vi "Install LabVIEW Support Legacy.vi"() -> ()   [LabVIEW 2020, in "LMH-LINX.lvlib"]
uses:
  LMH-LINX.lvlib
  Install LV Events.ctl
  Target Management/Install LV Data.ctl
  Target Management/Target Info.ctl
  Target Management/NIC Info.ctl
  Target Management/NIC Mode.ctl
  Target Management/Status FGV States.ctl
  <vilib>/Platform/browser.llb/Open URL in Default Browser (path).vi
  Toolbox/LMH-Toolbox.lvlib
panel:
  in  "Finish":bool
  in  "Example":bool
  in  "Install":bool
  in  "Password":string="raspberry"
  in  "Username":string="pi"
  in  "Hostname or IP":string="raspberrypi"
  out "Live Status":string
  in  "View Log":bool
  out "EULA Link":string="here"
  in  "Connect":bool
  out "Event Handler Iterations":i32
  out "Detailed Log":string
  out "Status Log":string
  out "Error Out":errorcluster
  # "LINX\nInstall LabVIEW Suport Wizard"
  # "This wizard will install LabVIEW support on BeagleBone Black or Raspberry Pi 2.\n\n1. Ensure the target is powered on, connected to this computer, and that the target has internet access.\n2. Enter the target's hostname or IP address.\n3. Enter the username and password for an account with sudo privileges on the target.\n          BBB defaults to 'root' and no password.\n          RPI2 running Raspbian defaults to 'pi' and 'raspberry'."
  # "The software installed by this wizard may be deployed on your hardware targets solely for your personal, \nnon-commercial use. Software is provided AS IS and with NO EXPRESS OR IMPLIED WARRANTIES.  \nThe full terms of the license can be found         ."
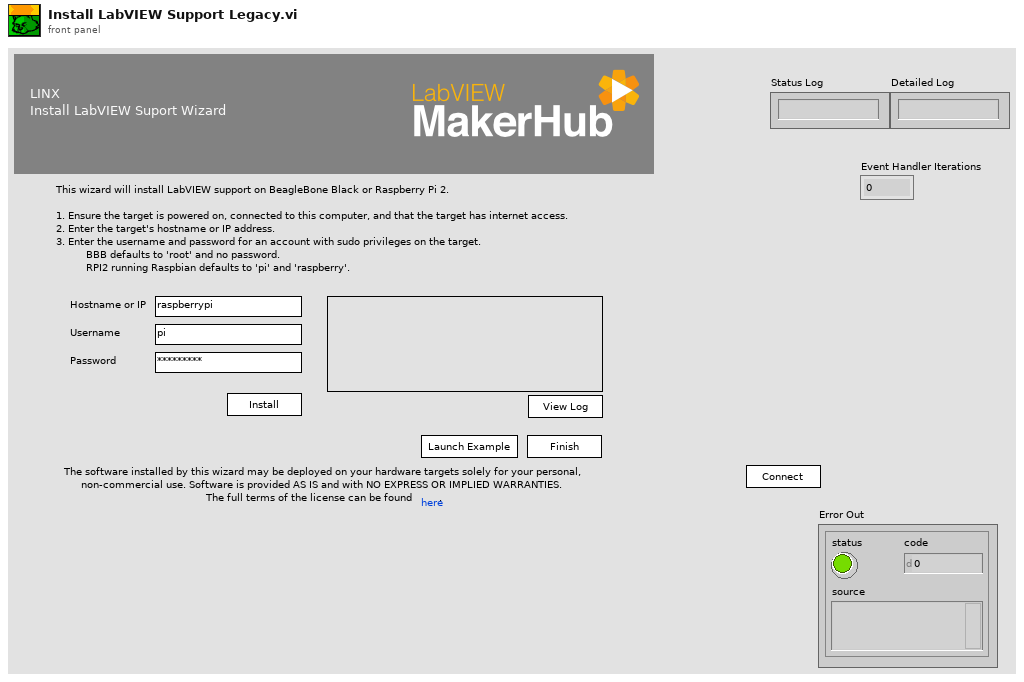
[diagram p1: front panel]
types:
  T1 = typedef "LMH-LINX.lvlib/Install LV Data.ctl" = cluster{"SSH Session":refnum<k1>, "Status Log":string, "Detailed Log":string, "Credentials":cluster{"Hostname or IP":string, "Username":string, "Password":string}, "Target Info":T2, "Reboot Required?":bool}
  T2 = typedef "LMH-LINX.lvlib/Target Info.ctl" = cluster{"OS Version":string, "CPU":string, "Systemd Version":string, "Internet Access":bool, "Device Type":string, "LV Installed Ver":string, "LV Available Ver":string, "LV Upgrade Available":bool, "Hostname":string, "NIC Info":T3[]}
  T3 = typedef "LMH-LINX.lvlib/NIC Info.ctl" = cluster{"Name":string, "NIC Mode":T4, "Configured":bool, "Config IP address":string, "Config Subnet mask":string, "Config Network":string, "Config gateway":string, "Wifi":bool, "SSID":string, "Password":string, "Configuration":string, "Current IP address":string, "Current Subnet mask":string, "Current gateway":string, "Current Network":string}
  T4 = typedef "LMH-LINX.lvlib/NIC Mode.ctl" = enum16{"DHCP", "Static", "Loopback"}
  T5 = typedef "LMH-LINX.lvlib/Install LV Events.ctl" = enum16{"Idle", "Connect", "Interrogate Device", "Pre Install", "Add MakerHub Feed", "Update Package Index", "Install LV", "Start LV", "Launch Example", "View Log", "Exit", "Update Hostname", "Menu: Target", "Menu: Install Software", "Menu: Network Settings", "Menu: Target Info", "NIC Select Change", "Menu: Network Settings Save", "Menu: Network Settings Cancel", "Menu: Cancel All"}
  T6 = typedef "LMH-LINX.lvlib/Status FGV States.ctl" = enum16{"Init", "Append", "Append History Only", "Set", "Get"}
  T7 = typedef "LMH-LINX.lvlib/Target Compatibility Warnings.ctl" = cluster{"Warning?":bool, "Details":string, "Help URL":string, "Fix It Button Name":string, "Fix It VI Ref":refnum<vi>}
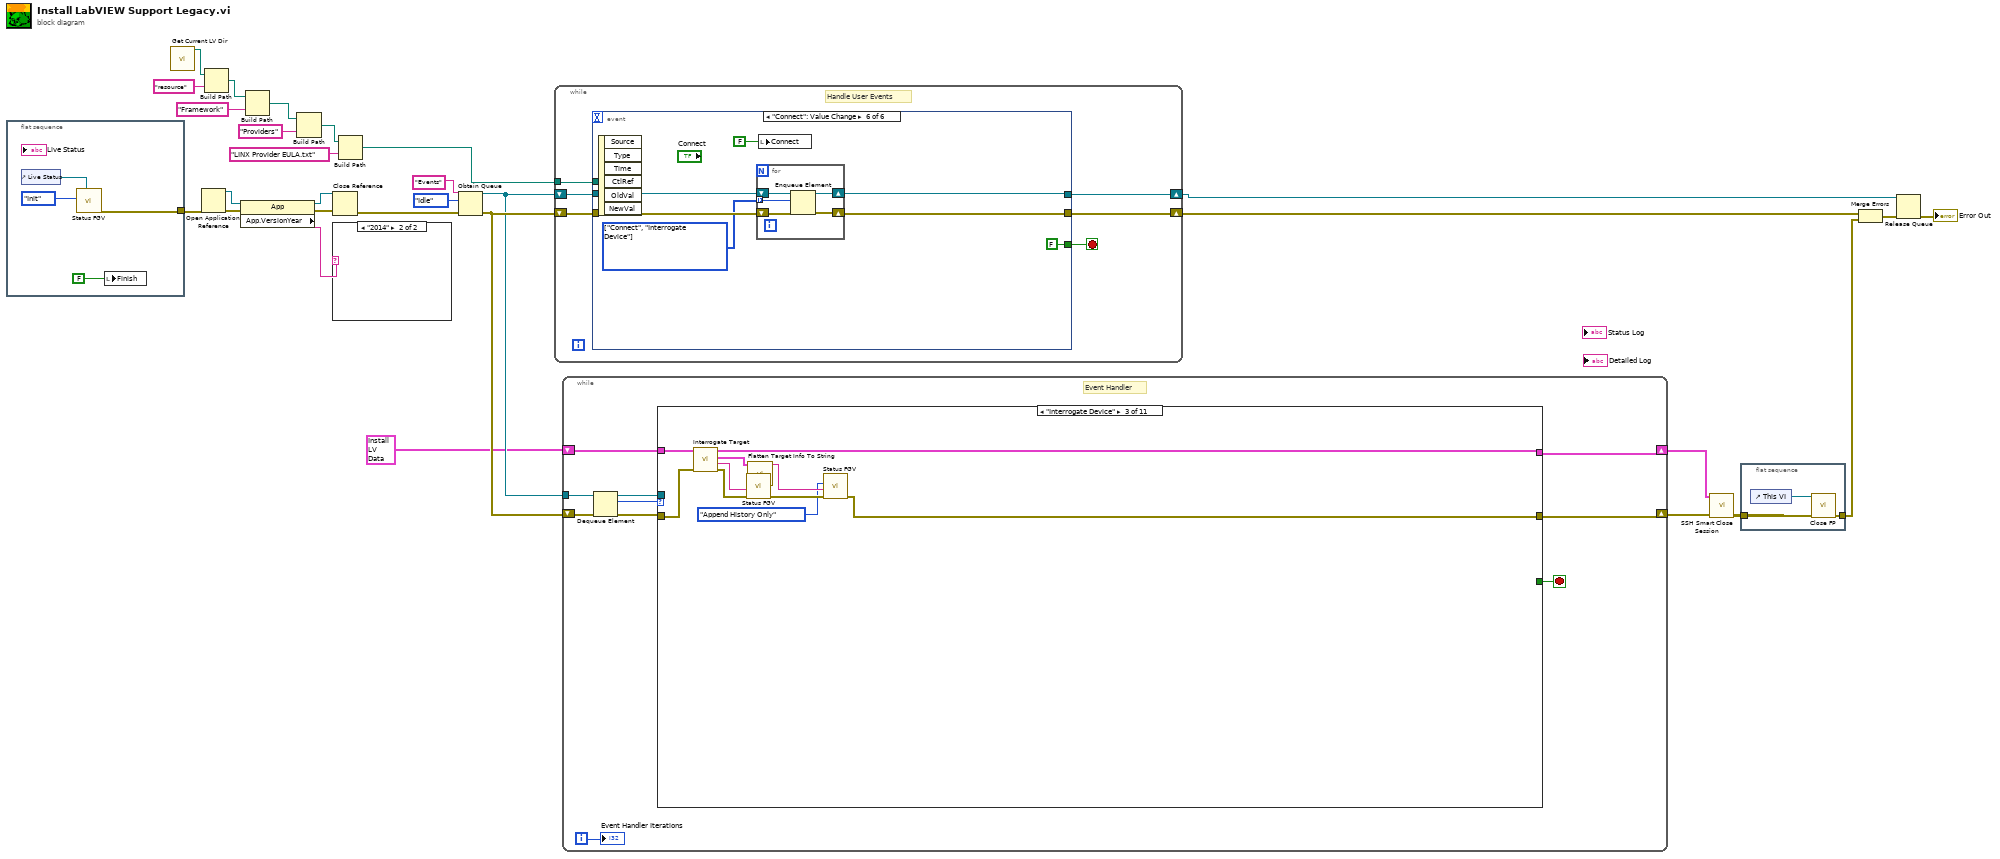
[diagram p0: block diagram]
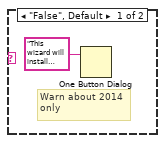
[diagram p2: hidden frame]
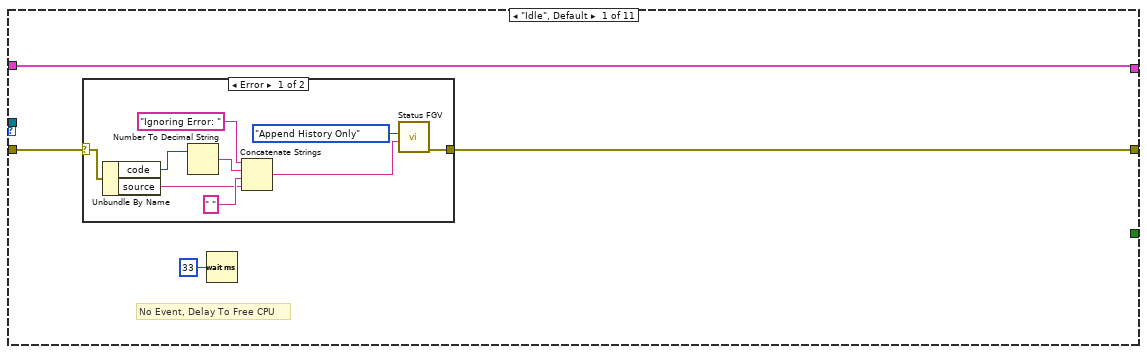
[diagram p3: hidden frame]
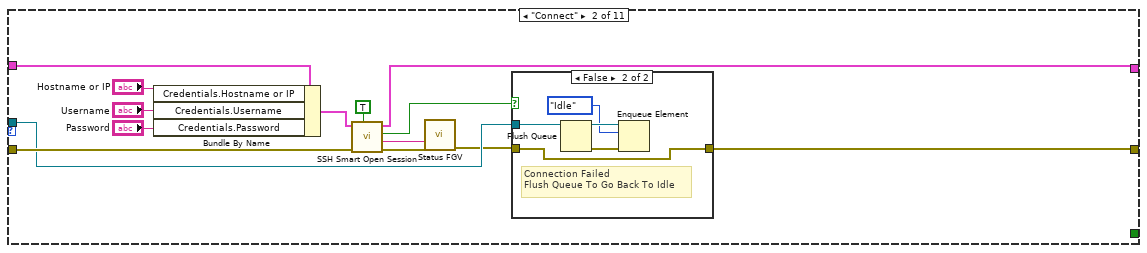
[diagram p5: hidden frame]
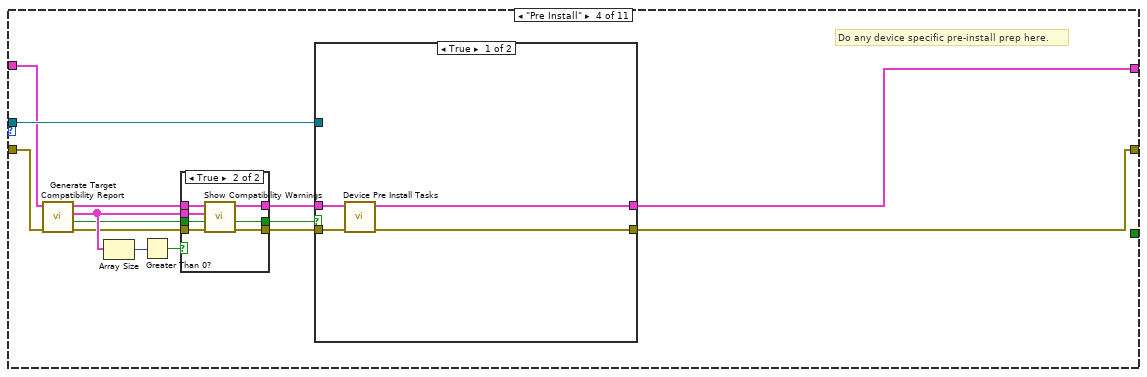
[diagram p7: hidden frame]
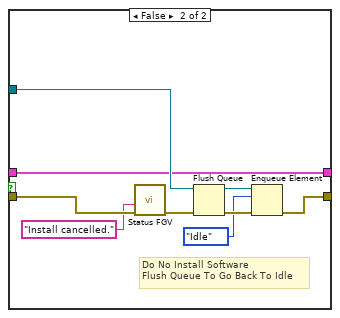
[diagram p8: hidden frame]
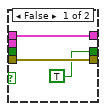
[diagram p9: hidden frame]
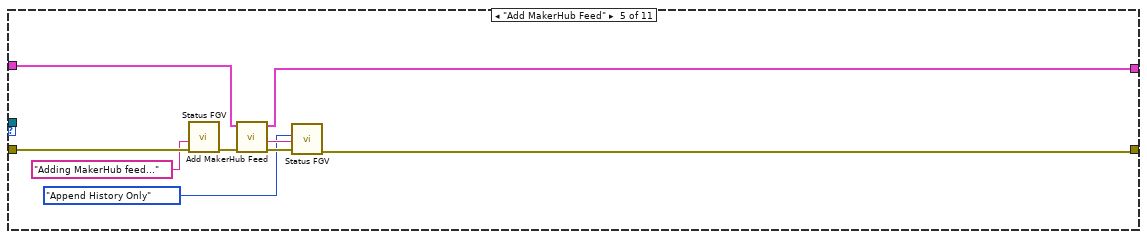
[diagram p10: hidden frame]
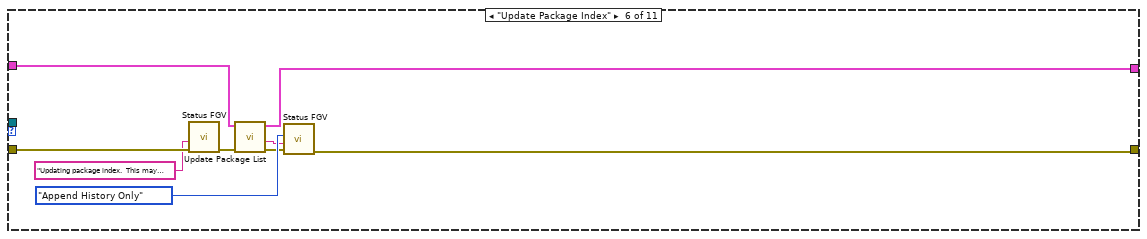
[diagram p11: hidden frame]
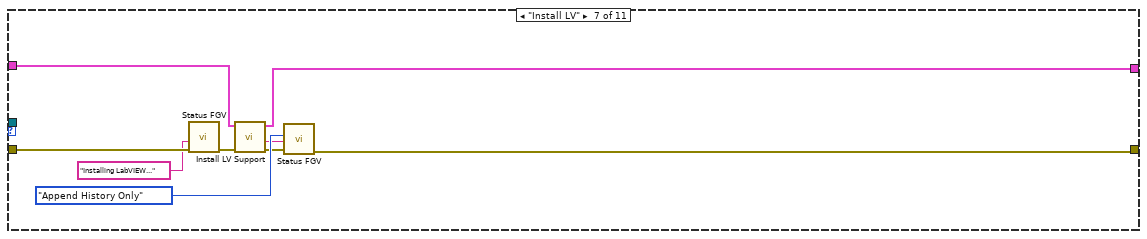
[diagram p12: hidden frame]
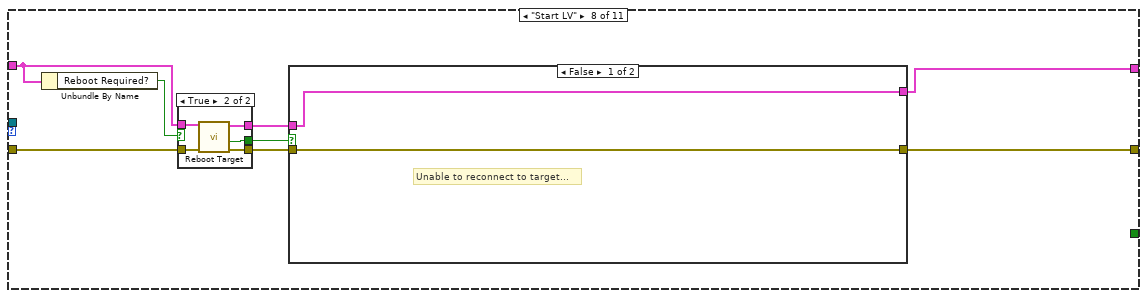
[diagram p13: hidden frame]
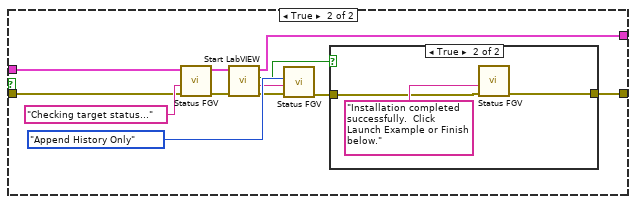
[diagram p14: hidden frame]
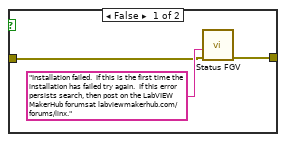
[diagram p15: hidden frame]
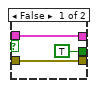
[diagram p16: hidden frame]
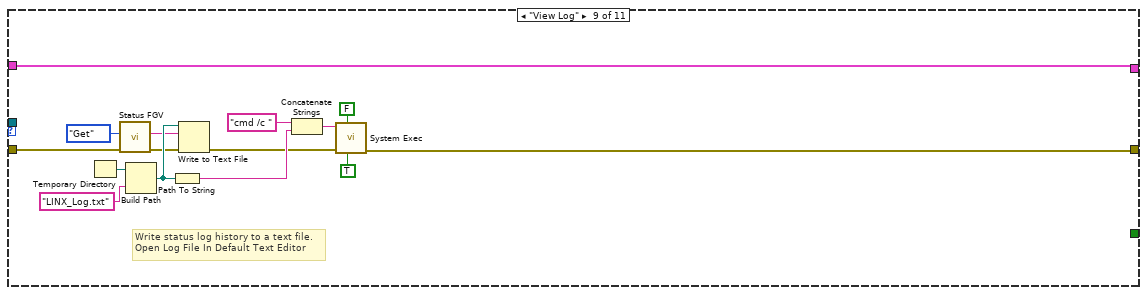
[diagram p17: hidden frame]
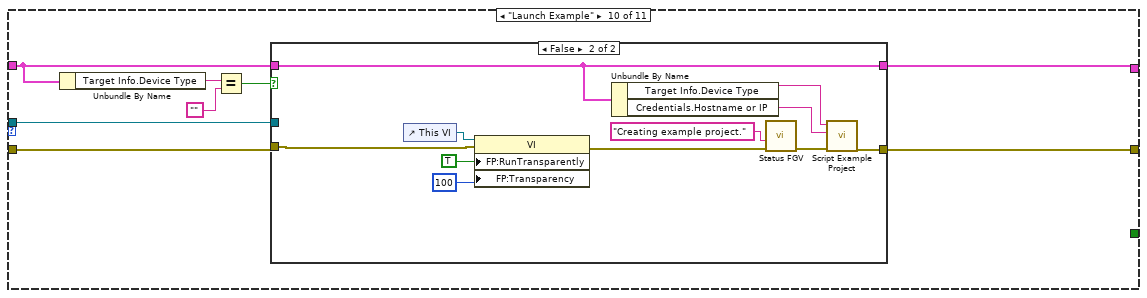
[diagram p18: hidden frame]
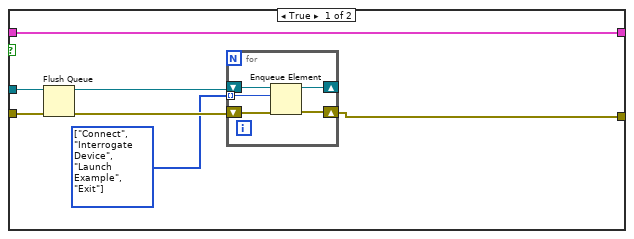
[diagram p19: hidden frame]
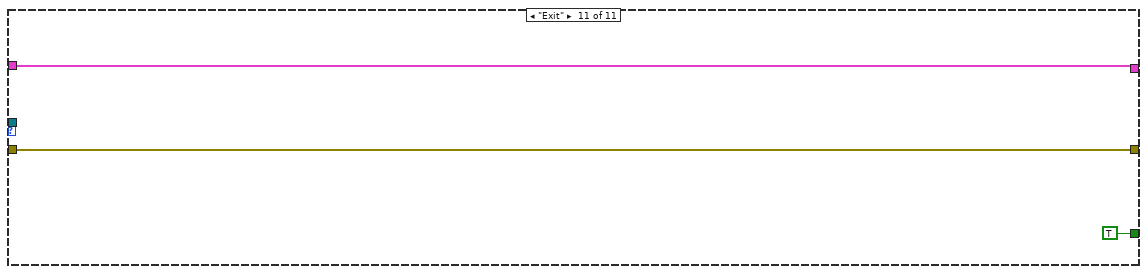
[diagram p20: hidden frame]
diagram:
  n1 = flat-sequence {
    tunnel: [w30] -> w6
    frame #0 {
      n2 = control-ref of="Live Status"() -> (w32:refnum<vi>)
      n3 = call "Status FGV.vi"("Live Status Ref"=w32, "Status FGV State"=Status_FGV_States."Init") -> ("Error Out"=w30:errorcluster)  [unwired: 7 in, 2 out]
      n4 = local write "Finish"(FALSE ("Stop Button")) -> ()
    }
  }
  n5 = call "Get Current LV Dir.vi"() -> ("This LV Directory"=w29:path)  [unwired: 10 in, 1 out]
  n6 = Open Application Reference(8:w6) -> (0:w19:errorcluster, 3:w16:refnum<vi>)  [unwired: 3 in]
  n7 = Build Path(base path=w29, name or relative path="resource") -> (appended path=w22:path)
  n8 = property class="App"(reference=w16, error in=w19) -> (reference out=w17:refnum<vi>, error out=w18:errorcluster, "App.VersionYear"=w20:string)
  n9 = Build Path(base path=w22, name or relative path="Framework") -> (appended path=w23:path)
  n10 = Build Path(base path=w23, name or relative path="Providers") -> (appended path=w24:path)
  n11 = Close Reference(reference=w17, error in (no error)=w18) -> (error out=w14:errorcluster)
  n12 = case shown="\"2014\"" w20 {
    frame "False", Default {
      # "Warn about 2014\nonly"
      n13 = One Button Dialog(message="This wizard will install LabVIEW 2014 support to the target device.  \nYou will only be able to connect to and use the device from LabVIEW 2014.") -> ()  [unwired: 1 in, 1 out]
    }
    frame "2014" {
    }
  }
  n14 = Build Path(base path=w24, name or relative path="LINX Provider EULA.txt") -> (appended path=w21:path)
  n15 = Obtain Queue(name (unnamed)="Events", element data type=Install_LV_Events."Idle" ("Install LV Support State"), error in (no error)=w14) -> (queue out=w12:refnum<queue>, error out=w13:errorcluster)  [unwired: 2 in, 1 out]
  n16 = while {
    shift-right: [w39] -> w2
    shift-left: w13 -> [w40]
    tunnel: w21 -> [w37]
    shift-right: [w36] -> w8
    shift-left: w12 -> [w35]
    stop <- w38 stop-if-true
    # "Handle User Events"
    n17 = event shown="[5] \"Connect\": Value Change" {
      selector: _ -> [_ _ _ _ _ _]
      dyn-events: _ -> [_ _ _ _ _ _]
      timeout: _ -> [_ _ _ _ _ _]
      tunnel: [w45 w64 w72 w76 w81 w92] -> w39
      tunnel: w40 -> [w46 w65 w70 w77 w86 w91]
      tunnel: [FALSE TRUE FALSE FALSE TRUE FALSE] -> w38
      tunnel: w37 -> [_ _ w71 _ _ _]
      tunnel: [w43 w63 w68 w75 w82 w93] -> w36
      tunnel: w35 -> [w42 w62 w68 w74 w87 w94]
      event "Install": Value Change {
        w41 = T5[] [enum."Connect", enum."Interrogate Device", enum."Pre Install", enum."Add MakerHub Feed", enum."Update Package Index", enum."Install LV", enum."Start LV"] items=["Idle", "Connect", "Interrogate Device", "Pre Install", "Add MakerHub Feed", "Update Package Index", "Install LV", "Start LV", "Launch Example", "View Log", "Exit", "Update Hostname", "Menu: Target", "Menu: Install Software", "Menu: Network Settings", "Menu: Target Info", "NIC Select Change", "Menu: Network Settings Save", "Menu: Network Settings Cancel", "Menu: Cancel All"]
        n18 = event-data() -> ("NewVal"=w44:bool)  [unwired: 1 in]
        n19 = local write "Install"(FALSE ("Install")) -> ()
        n20 = case shown="True" w44 {
          tunnel: w46 -> [w50 w55]
          tunnel: [w50 w54] -> w45
          tunnel: [w49 w53] -> w43
          tunnel: w42 -> [w49 w52]
          tunnel: w41 -> [_ w51]
          frame False {
            # "Ignore Change \nto False"
          }
          frame True {
            n21 = for {
              shift-right: [w59] -> w54
              shift-left: w55 -> [w60]
              shift-right: [w58] -> w53
              shift-left: w52 -> [w57]
              tunnel: w51 -> [w56] mode=indexing
              n22 = Enqueue Element(queue=w57, element=w56, error in (no error)=w60) -> (queue out=w58:refnum<queue>, error out=w59:errorcluster)  [unwired: 1 in, 1 out]
            }
          }
        }
      }
      event "Finish": Value Change {
        n23 = event-data() -> ()  [unwired: 1 in, 6 out]
        n24 = local write "Finish"(FALSE ("Stop Button")) -> ()
        n25 = Enqueue Element(queue=w62, element=Install_LV_Events."Exit", error in (no error)=w65) -> (queue out=w63:refnum<queue>, error out=w64:errorcluster)  [unwired: 1 in, 1 out]
      }
      event "EULA Link": Mouse Up {
        n26 = event-data() -> ()  [unwired: 1 in, 1 out]
        n27 = call-poly <vilib>:"Open URL in Default Browser.vi"("error in (no error)"=w70, "path"=w71) -> ("error out"=w72:errorcluster)  [unwired: 4 in, 1 out]
      }
      event "View Log": Value Change {
        n28 = event-data() -> ()  [unwired: 1 in, 1 out]
        n29 = Enqueue Element(queue=w74, element=Install_LV_Events."View Log", error in (no error)=w77) -> (queue out=w75:refnum<queue>, error out=w76:errorcluster)  [unwired: 1 in, 1 out]
        n30 = local write "View Log"(FALSE ("View Log")) -> ()
      }
      event "Example": Value Change {
        n31 = event-data() -> ()  [unwired: 1 in, 6 out]
        n32 = Enqueue Element(queue=w87, element=Install_LV_Events."Launch Example" ("Install LV Support State"), error in (no error)=w86) -> (queue out=w83:refnum<queue>, error out=w84:errorcluster)  [unwired: 1 in, 1 out]
        n33 = local write "Example"(FALSE ("Launch Example")) -> ()
        n34 = Enqueue Element(queue=w83, element=Install_LV_Events."Exit" ("Install LV Support State"), error in (no error)=w84) -> (queue out=w82:refnum<queue>, error out=w81:errorcluster)  [unwired: 1 in, 1 out]
      }
      event "Connect": Value Change {
        w90 = T5[] [enum."Connect", enum."Interrogate Device"] items=["Idle", "Connect", "Interrogate Device", "Pre Install", "Add MakerHub Feed", "Update Package Index", "Install LV", "Start LV", "Launch Example", "View Log", "Exit", "Update Hostname", "Menu: Target", "Menu: Install Software", "Menu: Network Settings", "Menu: Target Info", "NIC Select Change", "Menu: Network Settings Save", "Menu: Network Settings Cancel", "Menu: Cancel All"]
        n35 = event-data() -> ()  [unwired: 1 in, 6 out]
        n36 = for {
          shift-right: [w100] -> w92
          shift-left: w91 -> [w101]
          shift-right: [w99] -> w93
          shift-left: w94 -> [w98]
          tunnel: w90 -> [w97] mode=indexing
          n37 = Enqueue Element(queue=w98, element=w97, error in (no error)=w101) -> (queue out=w99:refnum<queue>, error out=w100:errorcluster)  [unwired: 1 in, 1 out]
        }
        n38 = local write "Connect"(FALSE ("Interrogate")) -> ()
      }
    }
  }
  n39 = while {
    shift-right: [w110] -> w7
    shift-left: w13 -> [w108]
    tunnel: w12 -> [w109]
    shift-right: [w105] -> w1
    shift-left: T1 {"SSH Session"=refnum, "Status Log"="", "Detailed Log"="", "Credentials"={"Hostname or IP"="", "Username"="", "Password"=""}, "Target Info"={"OS Version"="", "CPU"="", "Systemd Version"="", "Internet Access"=FALSE, "Device Type"="", "LV Installed Ver"="", "LV Available Ver"="", "LV Upgrade Available"=FALSE, "Hostname"="", "NIC Info"=[]}, "Reboot Required?"=FALSE} ("Install LV Data") -> [w103]
    i -> [w104]
    stop <- w111 stop-if-true
    # "Event Handler"
    n40 = Dequeue Element(queue=w109, error in (no error)=w108) -> (queue out=w102:refnum<queue>, element=w106:T5, error out=w107:errorcluster)  [unwired: 1 in, 1 out]
    n41 = case shown="\"Interrogate Device\"" w106 {
      tunnel: [w112 w135 w146 w160 w195 w207 w216 w227 w263 w276 w302] -> w110
      tunnel: w107 -> [w113 w139 w155 w164 w201 w210 w219 w225 w258 w277 w302]
      tunnel: [_ _ _ _ _ _ _ _ _ _ TRUE] -> w111
      tunnel: [w114 w126 w147 w159 w193 w202 w211 w221 w261 w270 w301] -> w105
      tunnel: w103 -> [w114 w128 w148 w158 w194 w203 w212 w223 w261 w271 w301]
      tunnel: w102 -> [_ w136 _ w165 _ _ _ _ _ w272 _]
      frame "Idle", Default {
        # "No Event, Delay To Free CPU"
        n42 = case shown="Error" w113 {
          selector: w113 -> [w123 w125]
          tunnel: [w124 w125] -> w112
          frame Error {
            n43 = Unbundle By Name(w123) -> ("code"=w121:i32, "source"=w118:string)
            n44 = Number To Decimal String(number=w121) -> (decimal integer string=w120:string)  [unwired: 1 in]
            n45 = Concatenate Strings("Ignoring Error: " ("Status"), w120, " " ("string"), w118) -> (w117:string)
            n46 = call "Status FGV.vi"("Status"=w117, "Status FGV State"=Status_FGV_States."Append History Only") -> ("Error Out"=w124:errorcluster)  [unwired: 7 in, 2 out]
          }
          frame No Error {
          }
        }
        n47 = Wait (ms)(milliseconds to wait=u32 33) -> ()  [unwired: 1 out]
      }
      frame "Connect" {
        n48 = Bundle By Name(cluster=w128, "Credentials.Hostname or IP"="Hostname or IP", "Credentials.Username"="Username", "Credentials.Password"="Password") -> (w127:T1)
        n49 = call "SSH Smart Open Session.vi"("Force Reconnect?"=TRUE, "Error In"=w139, "Install LV Data in"=w127) -> ("Error Out"=w134:errorcluster, "Status"=w132:string, "Connected?"=w137:bool, "Install LV Data out"=w126:T1)  [unwired: 5 in]
        n50 = call "Status FGV.vi"("Error In"=w134, "Status"=w132) -> ("Error Out"=w133:errorcluster)  [unwired: 7 in, 2 out]
        n51 = case shown="False" w137 {
          tunnel: w136 -> [_ w145]
          tunnel: w133 -> [w140 w141]
          tunnel: [w140 w141] -> w135
          frame True {
          }
          frame False {
            # "Connection Failed\nFlush Queue To Go Back To Idle"
            n52 = Flush Queue(queue=w145) -> (queue out=w143:refnum<queue>, error out=w144:errorcluster)  [unwired: 1 in, 1 out]
            n53 = Enqueue Element(queue=w143, element=Install_LV_Events."Idle", error in (no error)=w144) -> ()  [unwired: 1 in, 3 out]
          }
        }
      }
      frame "Interrogate Device" {
        n54 = call "Interrogate Target.vi"("Error In"=w155, "Install LV Data"=w148) -> ("Error Out"=w154:errorcluster, "Status"=w153:string, "Target Info"=w152:T2, "Install LV Data"=w147:T1)  [unwired: 6 in]
        n55 = call "Status FGV.vi"("Error In"=w154, "Status"=w153) -> ("Error Out"=w150:errorcluster)  [unwired: 7 in, 2 out]
        n56 = call "Flatten Target Info To String.vi"("Target Info"=w152) -> ("Target Info String"=w151:string)  [unwired: 10 in]
        n57 = call "Status FGV.vi"("Error In"=w150, "Status"=w151, "Status FGV State"=Status_FGV_States."Append History Only") -> ("Error Out"=w146:errorcluster)  [unwired: 6 in, 2 out]
      }
      frame "Pre Install" {
        # "Do any device specific pre-install prep here."
        n58 = call "Generate Target Compatibility Report.vi"("Error In"=w164, "Install LV Data"=w158) -> ("Error Out"=w161:errorcluster, "Can Continue?"=w162:bool, "Warnings"=w163:T7[], "Install LV Data"=w157:T1)  [unwired: 6 in]
        n59 = Array Size(array=w163) -> (size(s)=w169:i32)
        n60 = Greater Than 0?(x=w169) -> (x > 0?=w168:bool)
        n61 = case shown="True" w168 {
          tunnel: [w185 w192] -> w167
          tunnel: [TRUE ("Continue?") w191] -> w166
          tunnel: w161 -> [w185 w190]
          tunnel: w163 -> [_ w189]
          tunnel: w162 -> [_ w188]
          tunnel: w157 -> [w183 w187]
          tunnel: [w183 w186] -> w156
          frame False {
          }
          frame True {
            n62 = call "Show Compatibility Warnings.vi"("Error In"=w190, "Can Continue?"=w188, "Warnings"=w189, "Install LV Data"=w187) -> ("Error Out"=w192:errorcluster, "Continue?"=w191:bool, "Install LV Data"=w186:T1)  [unwired: 4 in, 1 out]
          }
        }
        n63 = case shown="True" w166 {
          tunnel: w167 -> [w173 w179]
          tunnel: [w172 w175] -> w160
          tunnel: w165 -> [_ w177]
          tunnel: [w171 w174] -> w159
          tunnel: w156 -> [w170 w174]
          frame True {
            n64 = call "Device Pre Install Tasks.vi"("Error In"=w173, "Install LV Data"=w170) -> ("Error Out"=w172:errorcluster, "Install LV Data"=w171:T1)  [unwired: 8 in]
          }
          frame False {
            # "Do No Install Software\nFlush Queue To Go Back To Idle"
            n65 = call "Status FGV.vi"("Error In"=w179, "Status"="Install cancelled.") -> ("Error Out"=w176:errorcluster)  [unwired: 7 in, 2 out]
            n66 = Flush Queue(queue=w177, error in (no error)=w176) -> (queue out=w181:refnum<queue>, error out=w182:errorcluster)  [unwired: 1 out]
            n67 = Enqueue Element(queue=w181, element=Install_LV_Events."Idle", error in (no error)=w182) -> (error out=w175:errorcluster)  [unwired: 1 in, 2 out]
          }
        }
      }
      frame "Add MakerHub Feed" {
        n68 = call "Status FGV.vi"("Error In"=w201, "Status"="Adding MakerHub feed...") -> ("Error Out"=w200:errorcluster)  [unwired: 7 in, 2 out]
        n69 = call "Add MakerHub Feed.vi"("Error In"=w200, "Install LV Data"=w194) -> ("Error Out"=w198:errorcluster, "Log"=w197:string, "Install LV Data"=w193:T1)  [unwired: 7 in]
        n70 = call "Status FGV.vi"("Error In"=w198, "Status"=w197, "Status FGV State"=Status_FGV_States."Append History Only") -> ("Error Out"=w195:errorcluster)  [unwired: 6 in, 2 out]
      }
      frame "Update Package Index" {
        n71 = call "Status FGV.vi"("Error In"=w210, "Status"="Updating package index.  This may take over 30 seconds depending on your internet speed...") -> ("Error Out"=w206:errorcluster)  [unwired: 7 in, 2 out]
        n72 = call "Update Package List.vi"("Error In"=w206, "Install LV Data"=w203) -> ("Error Out"=w205:errorcluster, "Log"=w204:string, "Install LV Data"=w202:T1)  [unwired: 7 in]
        n73 = call "Status FGV.vi"("Error In"=w205, "Status"=w204, "Status FGV State"=Status_FGV_States."Append History Only") -> ("Error Out"=w207:errorcluster)  [unwired: 6 in, 2 out]
      }
      frame "Install LV" {
        n74 = call "Status FGV.vi"("Error In"=w219, "Status"="Installing LabVIEW...") -> ("Error Out"=w213:errorcluster)  [unwired: 7 in, 2 out]
        n75 = call "Install LV Support.vi"("Error In"=w213, "Install LV Data"=w212) -> ("Error Out"=w215:errorcluster, "Log"=w214:string, "Install LV Data"=w211:T1)  [unwired: 7 in]
        n76 = call "Status FGV.vi"("Error In"=w215, "Status"=w214, "Status FGV State"=Status_FGV_States."Append History Only") -> ("Error Out"=w216:errorcluster)  [unwired: 6 in, 2 out]
      }
      frame "Start LV" {
        n77 = Unbundle By Name(w223) -> ("Reboot Required?"=w226:bool)
        n78 = case shown="True" w226 {
          tunnel: w225 -> [w248 w254]
          tunnel: [w248 w253] -> w224
          tunnel: w223 -> [w249 w252]
          tunnel: [w249 w251] -> w222
          tunnel: [TRUE ("Connected?") w250] -> w220
          frame False {
          }
          frame True {
            n79 = call "Reboot Target.vi"("Error In"=w254, "Install LV Data"=w252) -> ("Error Out"=w253:errorcluster, "Connected?"=w250:bool, "Install LV Data"=w251:T1)  [unwired: 7 in]
          }
        }
        n80 = case shown="False" w220 {
          tunnel: [w229 w235] -> w227
          tunnel: w224 -> [w229 w234]
          tunnel: w222 -> [w228 w233]
          tunnel: [w228 w232] -> w221
          frame False {
            # "Unable to reconnect to target..."
          }
          frame True {
            n81 = call "Status FGV.vi"("Error In"=w234, "Status"="Checking target status...") -> ("Error Out"=w238:errorcluster)  [unwired: 7 in, 2 out]
            n82 = call "Start LabVIEW.vi"("Error In"=w238, "Install LV Data"=w233) -> ("Error Out"=w237:errorcluster, "Log"=w236:string, "LV Running?"=w230:bool, "Install LV Data"=w232:T1)  [unwired: 6 in]
            n83 = call "Status FGV.vi"("Error In"=w237, "Status"=w236, "Status FGV State"=Status_FGV_States."Append History Only") -> ("Error Out"=w231:errorcluster)  [unwired: 6 in, 2 out]
            n84 = case shown="True" w230 {
              tunnel: [w243 w245] -> w235
              tunnel: w231 -> [w241 w244]
              frame False {
                n85 = call "Status FGV.vi"("Error In"=w241, "Status"="Installation failed.  If this is the first time the installation has failed try again.  If this error persists search, then post on the LabVIEW MakerHub forumsat labviewmakerhub.com/forums/linx.") -> ("Error Out"=w243:errorcluster)  [unwired: 7 in, 2 out]
              }
              frame True {
                n86 = call "Status FGV.vi"("Error In"=w244, "Status"="Installation completed successfully.  Click Launch Example or Finish below.") -> ("Error Out"=w245:errorcluster)  [unwired: 7 in, 2 out]
              }
            }
          }
        }
      }
      frame "View Log" {
        # "Write status log history to a text file.\nOpen Log File In Default Text Editor"
        n87 = Temporary Directory() -> (w269:path)
        n88 = call "Status FGV.vi"("Error In"=w258, "Status FGV State"=Status_FGV_States."Get") -> ("Error Out"=w257:errorcluster, "History"=w255:string)  [unwired: 7 in, 1 out]
        n89 = Build Path(base path=w269, name or relative path="LINX_Log.txt") -> (appended path=w260:path)
        n90 = Path To String(path=w260) -> (string=w264:string)
        n91 = Write to Text File(file (use dialog)=w260, text=w255, error in=w257) -> (error out=w259:errorcluster)  [unwired: 1 in, 2 out]
        n92 = Concatenate Strings("cmd /c " ("command line"), w264) -> (w267:string)
        n93 = call <vilib>:"System Exec.vi"("run minimized? (F)"=TRUE, "wait until completion? (T)"=FALSE, "error in (no error)"=w259, "command line"=w267) -> ("error out"=w263:errorcluster)  [unwired: 4 in, 3 out]
      }
      frame "Launch Example" {
        n94 = Unbundle By Name(w271) -> ("Target Info.Device Type"=w275:string)
        n95 = Equal?(x=w275, y="") -> (x = y?=w274:bool)
        n96 = case shown="False" w274 {
          tunnel: w277 -> [w284 w295]
          tunnel: [w279 w293] -> w276
          tunnel: w271 -> [w278 w290]
          tunnel: w272 -> [w283 _]
          tunnel: [w278 w290] -> w270
          frame True {
            w280 = T5[] [enum."Connect", enum."Interrogate Device", enum."Launch Example", enum."Exit"] items=["Idle", "Connect", "Interrogate Device", "Pre Install", "Add MakerHub Feed", "Update Package Index", "Install LV", "Start LV", "Launch Example", "View Log", "Exit", "Update Hostname", "Menu: Target", "Menu: Install Software", "Menu: Network Settings", "Menu: Target Info", "NIC Select Change", "Menu: Network Settings Save", "Menu: Network Settings Cancel", "Menu: Cancel All"] ("remaining elements")
            n97 = Flush Queue(queue=w283, error in (no error)=w284) -> (queue out=w281:refnum<queue>, error out=w282:errorcluster)  [unwired: 1 out]
            n98 = for {
              shift-right: [w288] -> w279
              shift-left: w282 -> [w289]
              shift-right: [w287] -> _
              shift-left: w281 -> [w286]
              tunnel: w280 -> [w285] mode=indexing
              n99 = Enqueue Element(queue=w286, element=w285, error in (no error)=w289) -> (queue out=w287:refnum<queue>, error out=w288:errorcluster)  [unwired: 1 in, 1 out]
            }
          }
          frame False {
            n100 = control-ref of="This VI"() -> (w296:refnum<vi>)
            n101 = property class="VI"(reference=w296, error in=w295, "FP:RunTransparently"=TRUE ("Front Panel Window:Run VI Transparently"), "FP:Transparency"=u8 100 ("Front Panel Window:Transparency")) -> (error out=w294:errorcluster)  [unwired: 1 out]
            n102 = Unbundle By Name(w290) -> ("Target Info.Device Type"=w298:string, "Credentials.Hostname or IP"=w297:string)
            n103 = call "Status FGV.vi"("Error In"=w294, "Status"="Creating example project.") -> ("Error Out"=w299:errorcluster)  [unwired: 7 in, 2 out]
            n104 = call "Script Example Project.vi"("Error In"=w299, "Hostname or IP"=w297, "Device Name"=w298) -> ("Error Out"=w293:errorcluster)  [unwired: 8 in]
          }
        }
      }
      frame "Exit" {
      }
    }
    "Event Handler Iterations" <- w104
  }
  n105 = call "SSH Smart Close Session.vi"("Error In"=w7, "Install LV Data"=w1) -> ("Error Out"=w3:errorcluster)  [unwired: 8 in, 1 out]
  n106 = flat-sequence {
    tunnel: [w305] -> w5
    tunnel: w3 -> [w304]
    frame #0 {
      n107 = control-ref of="This VI"() -> (w306:refnum<vi>)
      n108 = call "Close FP.vi"("Error In"=w304, "VI Ref"=w306) -> ("Error Out"=w305:errorcluster)  [unwired: 9 in]
    }
  }
  n109 = Merge Errors(w2, w5) -> (w9:errorcluster)
  n110 = Release Queue(queue=w8, error in (no error)=w9) -> (error out=→"Error Out":errorcluster)  [unwired: 1 in, 2 out]
